vi "BioFeedback17(Queue).vi"(7 "Frames Per Second":dbl=30.0, 9 "Start Trial":bool, 11 "End Trial":bool, 12 "Data Directory":path=path "C:/Users/Tinggroup/Desktop/VRMuscleActivationVisualizer/LabviewFiles/Data/Test", 13 "File Name":string="Test") -> ()   [LabVIEW 2016]
uses:
  customSubVIs/Control 1.ctl
  <vilib>/Utility/file.llb/Write Delimited Spreadsheet (DBL).vi
  <vilib>/Waveform/WDTFileIO.llb/Export Waveforms To Spreadsheet File (1D).vi
  <vilib>/Utility/file.llb/Write Delimited Spreadsheet (I64).vi
  <vilib>/Utility/error.llb/DialogType.ctl
panel:
  out "error out 3":errorcluster
  out "Raw Trial Data Wfm 2":waveform(dbl)[](graph)
  out "Terminate":bool=TRUE
  out "Waveform":waveform(dbl)
  out "Notes":T1(array[cluster])
  in  "Mark":bool
  out "error out 2":errorcluster
  out "error out":errorcluster
  out "MVC Buffer Index":dbl=3.0
  in  "DisplayDataPath":path
  in  "FilteredDataPath":path
  in  "RawDataPath":path
  in  "MVC Number":dbl=1.0
  out "Save MVC":bool
  out "Display Buffer":dbl[][](array[numeric])
  out "Display Buffer Index":dbl=3.0
  out "FilteredTrialData Display Channel":waveform(dbl)(graph)
  out "Raw Trial Data Display Channel":waveform(dbl)(graph)
  out "EndProcessTic":u32
  out "StartProcessTic":u32
  out "EndRecordTic":u32
  out "startRecordTic":u32
  out "Start UI":timestamp
  out "UI Elapsed Time":u32
  out "End UI":timestamp
  out "Process Elapsed Time":u32
  out "Record Elapsed Time":u32
  out "FilteredTrialData":waveform(dbl)[](graph)
  out "FilteredAndRectified":waveform(dbl)[](graph) caption="Filtered and Rectified"
  out "FilteredDataArray":waveform(dbl)[](array[waveform])
  in  "DisplayChannel":dbl
  out "DisplayTrialData":T2
  out "DisplayValueByChannel":dbl[](array[numeric])
  out "MVCBufferSize":dbl
  in  "MVC Window Size (s)":dbl=0.5
  out "MVC Buffer":dbl[][](array[numeric])
  out "GetMaxStartTime":timestamp
  in  "SecondsToAcquireMax":dbl=3.0
  out "MVCArray":dbl[](array[numeric])
  out "RawTrialData":waveform(dbl)[](array[waveform])
  in  "UI Ampl Error Path":path=path "C:/Users/Tinggroup/Desktop/VRMuscleActivationVisualizer/VRBiofeedback_v2/assets/BiofeedbackAmplitudeError.txt"
  out "DisplayActivation":dbl
  out "Get MVC":bool
  in  "resetMax":bool
  in  "startGetMax":bool
  in  "Amplitude Error":dbl
  in  "UI Data Path":path=path "C:/Users/Tinggroup/Desktop/VRMuscleActivationVisualizer/VRBiofeedback_v2/assets/LeftEMGData.txt"
  in  "EMG Input Device\nProduct Type":string="USB-6009"
  out "DisplayBarActivation":dbl(slide) caption="Left" max=1.0 scale=0.0..100.0
  out "NormalizedSignal8":dbl[](graph)
  out "NormalizedSignal7":dbl[](graph)
  out "NormalizedSignal6":dbl[](graph)
  out "NormalizedSignal5":dbl[](graph)
  out "NormalizedSignal4":dbl[](graph)
  out "NormalizedSignal3":dbl[](graph)
  out "NormalizedSignal2":dbl[](graph)
  out "NormalizedSignal1":dbl[](graph)
  out "Raw Trial Data Wfm":waveform(dbl)[](graph)
  in  "UI Percent Path":path=path "C:/Users/Tinggroup/Desktop/VRMuscleActivationVisualizer/VRBiofeedback_v2/assets/BiofeedbackTargetPercentage.txt"
  in  "Target Percentage":dbl=10.0
  out "Trial In Progress":bool
  in  "Lower Cut-Off":dbl=20.0
  in  "Upper Cut-Off":dbl=300.0
  out "raw data":dynamicdata(graph)
  out "DisplayBufferSize":dbl
  out "Samples per frame":dbl
  out "Reset":bool=TRUE
  in  "Display Window Size (s)":dbl=0.5
  in  "Sample rate (Hz)":dbl=2000.0
  in  "End Program":bool
  # "Data To Be Saved (Not including Max Data)"
  # "Performance Metrics"
  # "Saving Trial Data"
  # "Small Window"
  # "Scale Max"
  # "Filter and Process Parameters"
  # "MVC Buffer"
  # "Set Target"
  # "Display Parameters"
  # "Changes are made instantly and cause moving average to reset to zero"
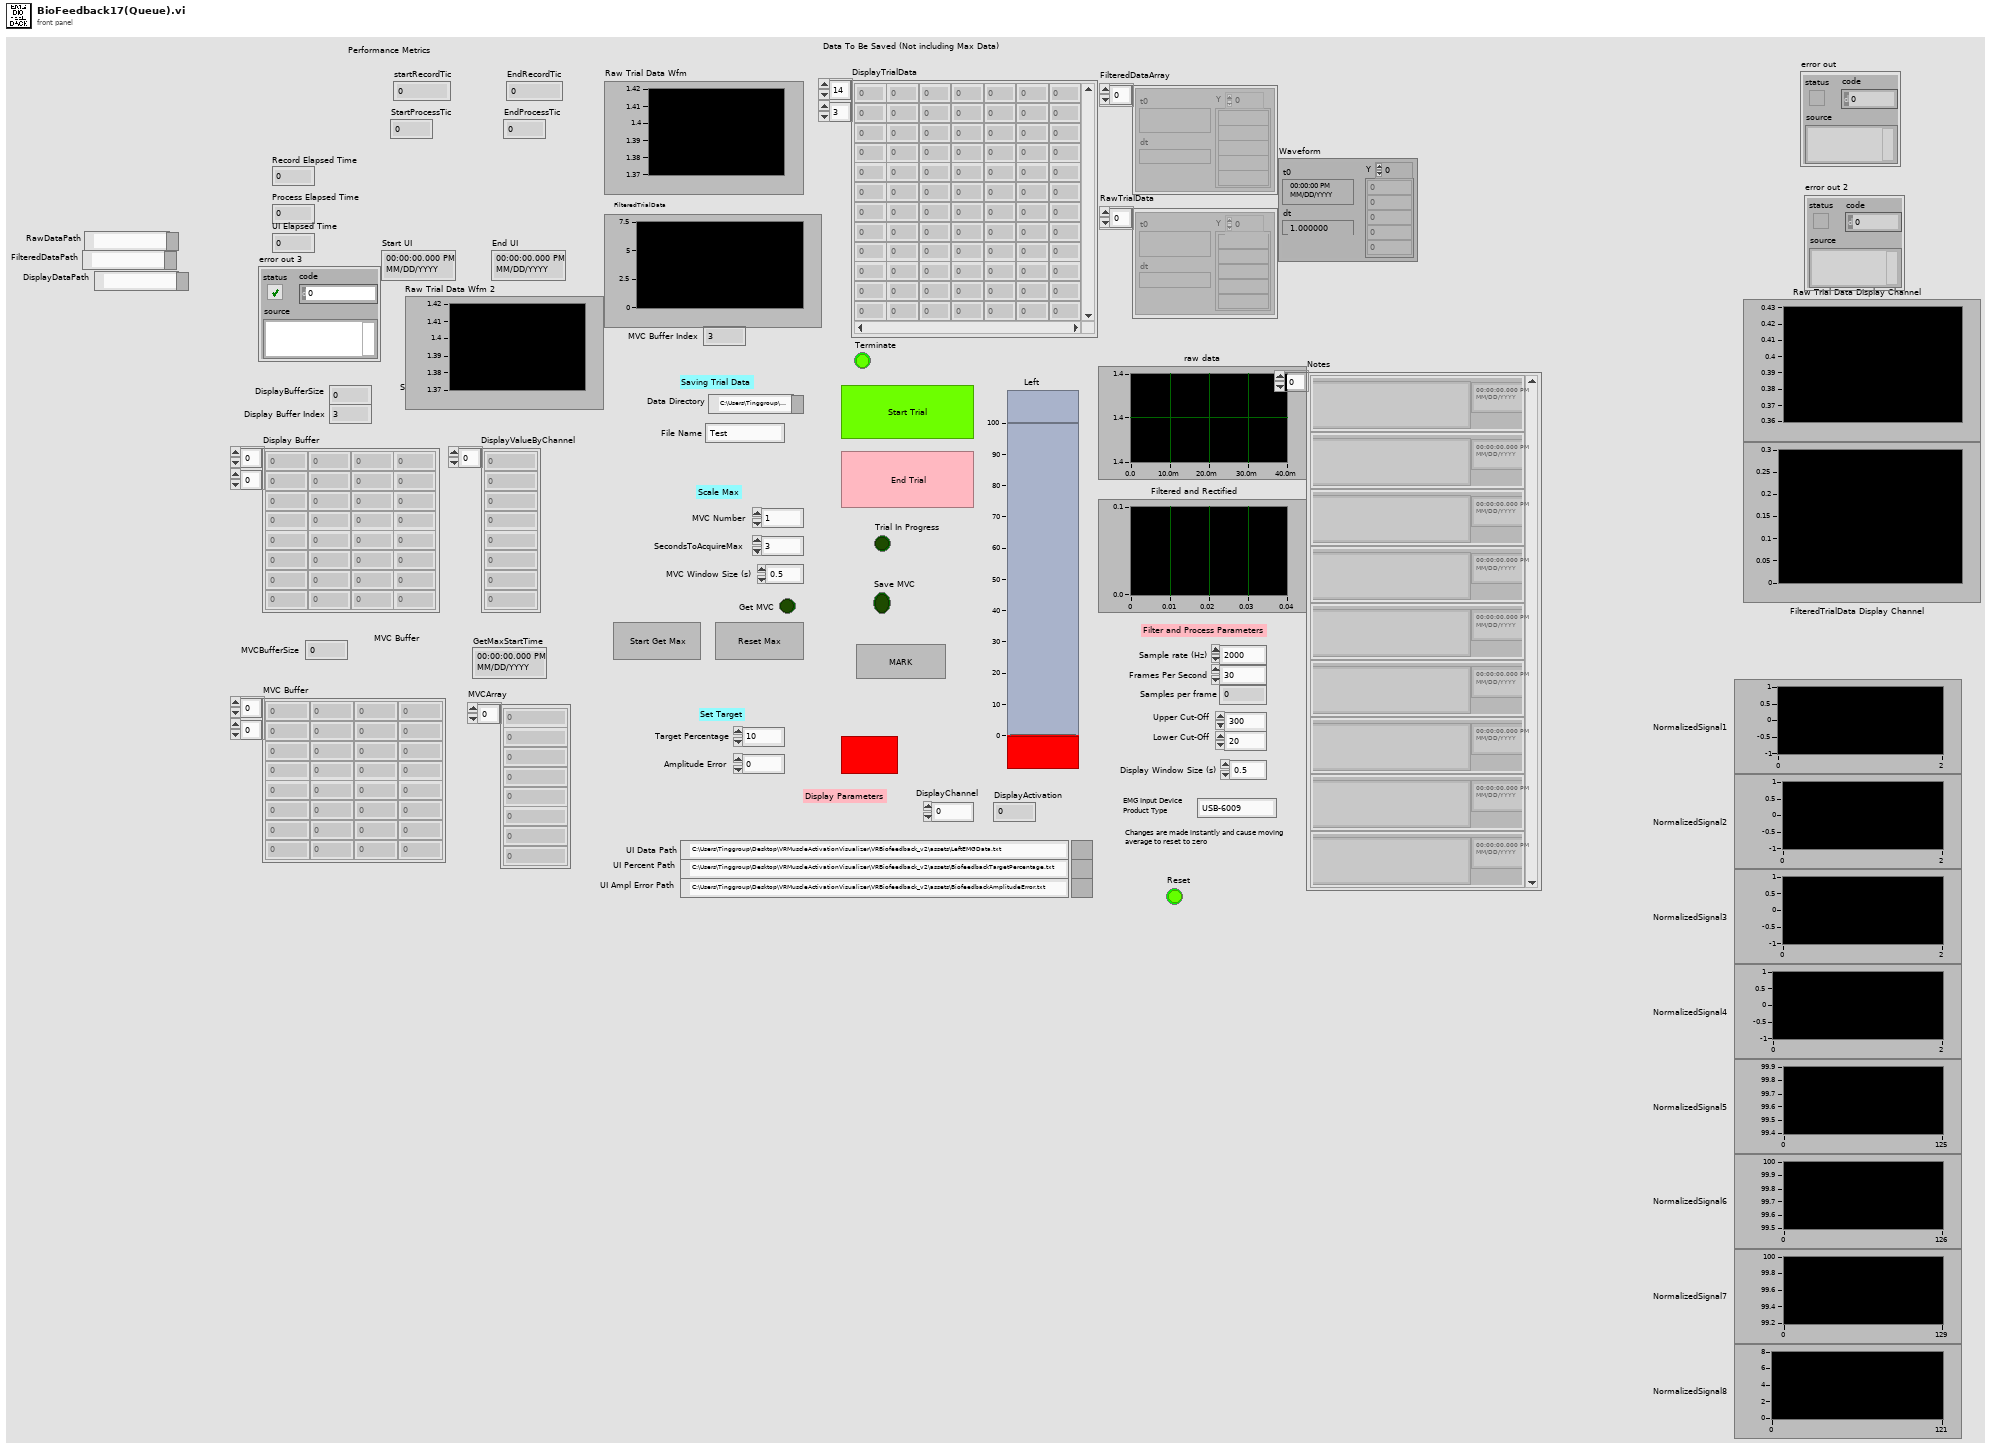
[diagram p1: front panel]
types:
  T1 = cluster{"Time Stamp":timestamp, "String":string}[]
  T2 = typedef "Control 1.ctl" = dbl[][]
  T3 = cluster{"seconds since 1Jan1904":timestamp, string}
  T4 = typedef "DialogType.ctl" = u16
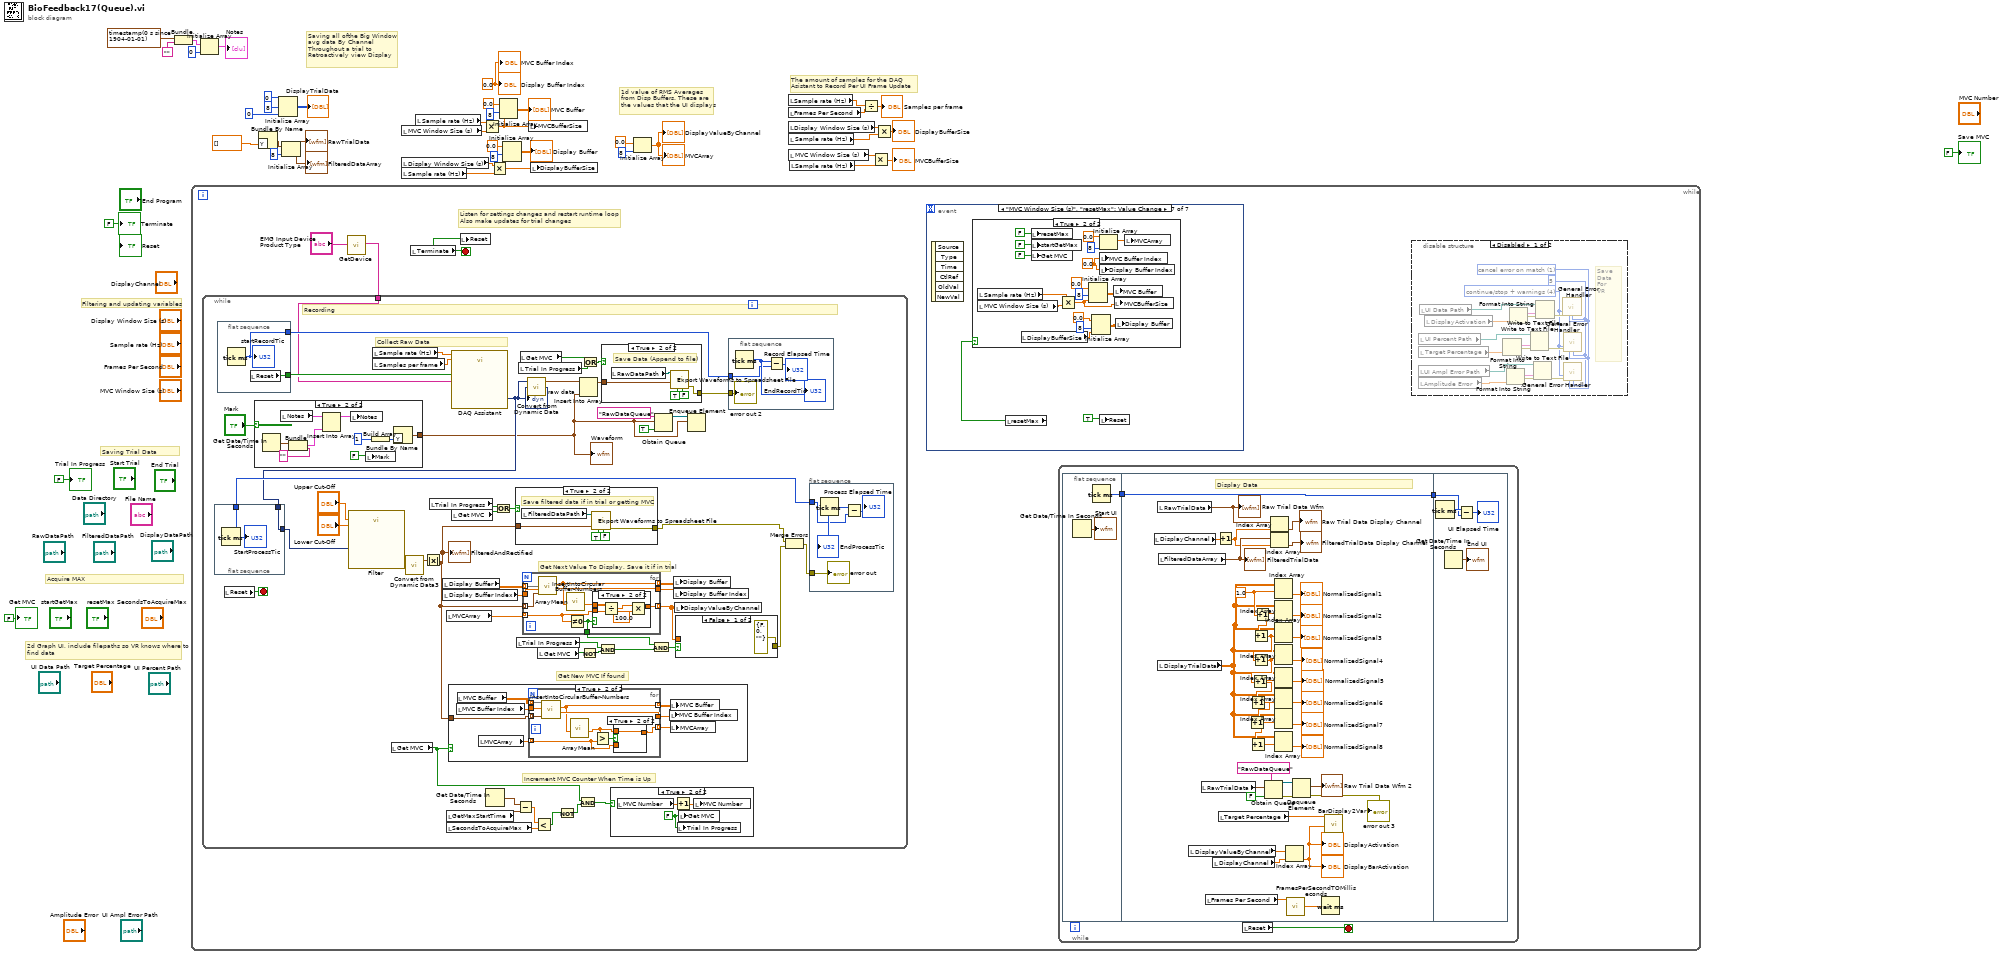
[diagram p0: block diagram]
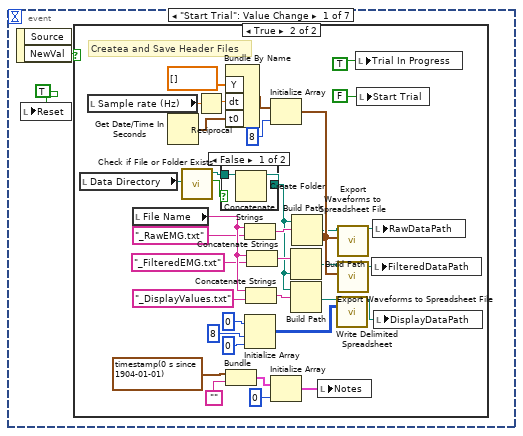
[diagram p3: hidden frame]
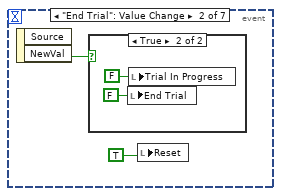
[diagram p6: hidden frame]
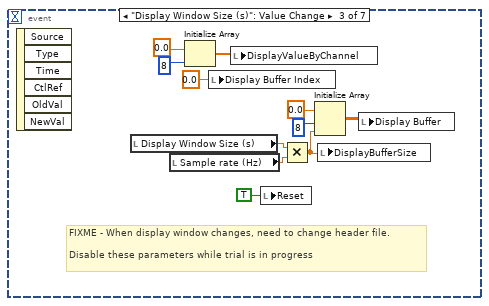
[diagram p8: hidden frame]
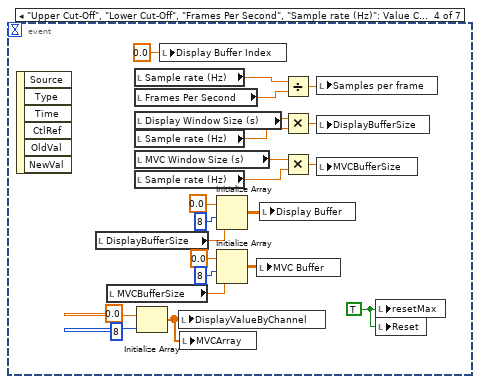
[diagram p9: hidden frame]
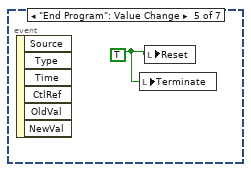
[diagram p10: hidden frame]
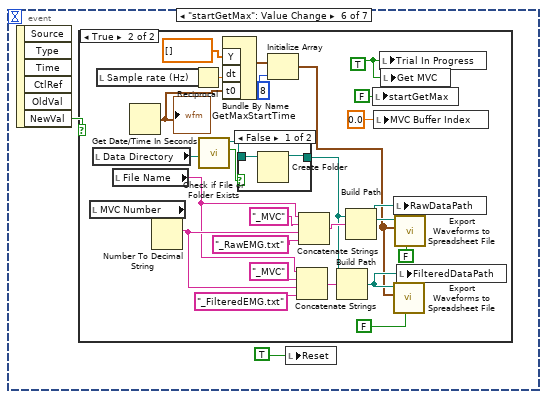
[diagram p11: hidden frame]
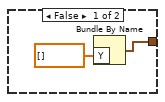
[diagram p15: hidden frame]
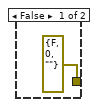
[diagram p16: hidden frame]
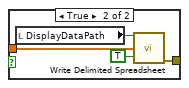
[diagram p17: hidden frame]
diagram:
  w13 = 0.0 ("Display Buffer Index")
  # "The amount of samples for the DAQ Asistant to Record Per UI Frame Update"
  # "Saving all ofthe Big Window \navg data By Channel\nThroughout a trial to \nRetroactively view Display"
  # "1d value of RMS Averages\nfrom Disp Buffers. These are\nthe values that the UI displays"
  # "Acquire MAX"
  # "Filtering and updating variables"
  # "Saving Trial Data"
  # "2d Graph UI, include filepaths so VR knows where to find data"
  n1 = Bundle(timestamp(0 s since 1904-01-01), "") -> (w12:cluster{timestamp, string})  [unwired: 1 in]
  n2 = while {
    stop <- w43 stop-if-true
    # "Listen for settings changes and restart runtime loop\nAlso make updates for trial changes"
    n3 = call "GetDevice.vi"("EMG Input Device\nProduct Type"="EMG Input Device\nProduct Type") -> ("DAQmx Device Name"=w45:tag)  [unwired: 10 in]
    n4 = while {
      tunnel: w45 -> [w247]
      stop <- w286 stop-if-true
      # "Recording"
      # "Collect Raw Data"
      # "Increment MVC Counter When Time is Up"
      # "Get New MVC If found"
      # "Get Next Value To Display, Save it if in trial"
      n5 = flat-sequence {
        tunnel: [w315] -> w258
        tunnel: [w314] -> w241
        tunnel: w240 -> [w314]
        frame #0 {
          n6 = Tick Count (ms)() -> (millisecond timer value=w315:u32)
          "StartProcessTic" <- w315
        }
      }
      n7 = flat-sequence {
        tunnel: [w303] -> w252
        tunnel: [w302] -> w251
        frame #0 {
          n8 = Tick Count (ms)() -> (millisecond timer value=w302:u32)
          "startRecordTic" <- w302
          n9 = local read "Reset"() -> (w303:bool)
        }
      }
      n10 = local read "Reset"() -> (w286:bool)
      n11 = case shown="True" "Mark" {
        tunnel: [w287 w290] -> w236
        frame False {
          n12 = Bundle By Name("Y"=dbl[] []) -> (w287:waveform(dbl))  [unwired: 1 in]
        }
        frame True {
          n13 = Get Date/Time In Seconds() -> (seconds since 1Jan1904=w296:timestamp)
          n14 = local read "Notes"() -> (w293:T1)
          n15 = Bundle("seconds since 1Jan1904"=w296, "") -> (w292:T3)  [unwired: 1 in]
          n16 = Insert Into Array(array=w293, new element=w292) -> (w294:T1)  [unwired: 1 in]
          n17 = local write "Notes"(w294) -> ()
          n18 = local write "Mark"(FALSE) -> ()
          n19 = Build Array(1) -> (w291:i32[])
          n20 = Bundle By Name("Y"=w291) -> (w290:waveform(i32))  [unwired: 1 in]
        }
      }
      "Waveform" <- w236
      n21 = call "Filter"("Lower Cut-Off"="Lower Cut-Off", "Upper Cut-Off"="Upper Cut-Off", "Signal"=w241) -> ("Filtered Signal"=w242:dynamicdata)  [unwired: 7 in, 1 out]
      n22 = local read "Sample rate (Hz)"() -> (w253:dbl)
      n23 = local read "Samples per frame"() -> (w254:dbl)
      n24 = local read "Get MVC"() -> (w279:bool)
      n25 = call "Convert from Dynamic Data3"("Dynamic Data Type"=w242) -> ("Array of Waveform"=w259:waveform(dbl)[])  [unwired: 3 in]
      n26 = Absolute Value(x=w259) -> (abs(x)=w274:waveform(dbl)[])
      "FilteredAndRectified" <- w274
      n27 = local read "Trial In Progress"() -> (w262:bool)
      n28 = local read "Display Buffer"() -> (w265:dbl[][])
      n29 = local read "Display Buffer Index"() -> (w266:dbl)
      n30 = local read "MVCArray"() -> (w269:dbl[])
      n31 = local read "GetMaxStartTime"() -> (w273:timestamp)
      n32 = local read "SecondsToAcquireMax"() -> (w270:dbl)
      n33 = case shown="True" w279 {
        tunnel: w274 -> [_ w328]
        frame False {
        }
        frame True {
          n34 = local read "MVC Buffer Index"() -> (w330:dbl)
          n35 = local read "MVC Buffer"() -> (w329:dbl[][])
          n36 = local read "MVCArray"() -> (w327:dbl[])
          n37 = for {
            tunnel: w329 -> [w339] mode=indexing
            tunnel: w330 -> [w331]
            tunnel: [w338] -> w324
            tunnel: w328 -> [w337] mode=indexing
            tunnel: w327 -> [w333] mode=indexing
            tunnel: [w332] -> w326 mode=indexing
            tunnel: [w334] -> w325 mode=indexing
            n38 = call "InsertIntoCircularBuffer-Numbers.vi"("NewElements"=w337, "StartIndex"=w331, "Buffer"=w339) -> ("New Start Index"=w338:dbl, "UpdatedBuffer"=w334:dbl[])  [unwired: 7 in]
            n39 = call "ArrayMean.vi"("Array"=w334) -> ("Mean"=w335:dbl)  [unwired: 10 in]
            n40 = Greater?(x=w335, y=w333) -> (0:w336:bool)
            n41 = case shown="True" w336 {
              tunnel: w335 -> [_ w341]
              tunnel: [w340 w341] -> w332
              tunnel: w333 -> [w340 _]
              frame False {
              }
              frame True {
              }
            }
          }
          n42 = local write "MVC Buffer Index"(w324) -> ()
          n43 = local write "MVC Buffer"(w325) -> ()
          n44 = local write "MVCArray"(w326) -> ()
        }
      }
      n45 = call "DAQ Assistant"("rate"=w253, "number of samples"=w254, "stop (F)"=w252, "device name"=w247) -> ("data"=w240:dynamicdata)  [unwired: 12 in, 3 out]
      "raw data" <- w240
      n46 = local read "Get MVC"() -> (w264:bool)
      n47 = Get Date/Time In Seconds() -> (seconds since 1Jan1904=w272:timestamp)
      n48 = Or(x=w262, y=w264) -> (x .or. y?=w263:bool)
      n49 = case shown="True" w263 {
        tunnel: w274 -> [_ w359]
        tunnel: [errorcluster {"status"=FALSE, "code"=0, "source"=""} ("error out") w358] -> w249
        frame False {
        }
        frame True {
          # "Save filtered data if in trial or getting MVC"
          n50 = local read "FilteredDataPath"() -> (w360:path)
          n51 = call-poly <vilib>:"Export Waveforms to Spreadsheet File.vi"("header? (write header:T)"=FALSE, "append to file? (new file:F)"=TRUE, "waveforms"=w359, "file path (dialog if empty)"=w360) -> ("error out"=w358:errorcluster)  [unwired: 6 in, 1 out]
        }
      }
      n52 = local read "Trial In Progress"() -> (w284:bool)
      n53 = Subtract(x=w272, y=w273) -> (x-y=w271:dbl)
      n54 = local read "Trial In Progress"() -> (w255:bool)
      n55 = local read "Get MVC"() -> (w256:bool)
      n56 = for {
        tunnel: w265 -> [w350] mode=indexing
        tunnel: w274 -> [w343] mode=indexing
        tunnel: w266 -> [w349]
        tunnel: [w347] -> w267 mode=indexing
        tunnel: [w348] -> w268
        tunnel: w269 -> [w345] mode=indexing
        tunnel: [w344] -> w278 mode=indexing
        tunnel: [w342] -> w281
        n57 = call "InsertIntoCircularBuffer-Numbers.vi"("NewElements"=w343, "StartIndex"=w349, "Buffer"=w350) -> ("New Start Index"=w348:dbl, "UpdatedBuffer"=w347:dbl[])  [unwired: 7 in]
        n58 = call "ArrayMean.vi"("Array"=w347) -> ("Mean"=w346:dbl)  [unwired: 10 in]
        n59 = Not Equal To 0?(x=w345) -> (x != 0?=w342:bool)
        n60 = case shown="True" w342 {
          tunnel: w346 -> [_ w355]
          tunnel: w345 -> [_ w356]
          tunnel: [0.0 w354] -> w344
          frame False {
          }
          frame True {
            n61 = Divide(x=w355, y=w356) -> (x/y=w353:dbl)
            n62 = Multiply(x=w353, y=100.0) -> (x*y=w354:dbl)
          }
        }
      }
      n63 = call "Convert from Dynamic Data"("Dynamic Data Type"=w240) -> ("Array of Waveform"=w244:waveform(dbl)[])  [unwired: 3 in]
      n64 = Less?(x=w271, y=w270) -> (x < y?=w275:bool)
      n65 = local read "Get MVC"() -> (w282:bool)
      n66 = Not(x=w275) -> (.not. x?=w276:bool)
      n67 = And(x=w279, y=w276) -> (x .and. y?=w277:bool)
      n68 = Insert Into Array(array=w244, new element=w236) -> (w243:waveform(dbl)[])  [unwired: 1 in]
      n69 = Not(x=w282) -> (.not. x?=w283:bool)
      n70 = Or(x=w256, y=w255) -> (x .or. y?=w257:bool)
      n71 = And(x=w284, y=w283) -> (x .and. y?=w285:bool)
      n72 = case shown="True" w257 {
        tunnel: w243 -> [_ w307]
        tunnel: [errorcluster {"status"=FALSE, "code"=0, "source"=""} ("error out") w305] -> w246
        frame False {
        }
        frame True {
          # "Save Data (Append to file)"
          n73 = local read "RawDataPath"() -> (w306:path)
          n74 = call-poly <vilib>:"Export Waveforms to Spreadsheet File.vi"("header? (write header:T)"=FALSE, "append to file? (new file:F)"=TRUE, "waveforms"=w307, "file path (dialog if empty)"=w306) -> ("error out"=w305:errorcluster)  [unwired: 6 in, 1 out]
        }
      }
      n75 = case shown="True" w277 {
        frame False {
        }
        frame True {
          w321 = FALSE ("Get MVC")
          n76 = local read "MVC Number"() -> (w322:dbl)
          n77 = Increment(x=w322) -> (x+1=w323:dbl)
          n78 = local write "Trial In Progress"(w321) -> ()
          n79 = local write "Get MVC"(w321) -> ()
          n80 = local write "MVC Number"(w323) -> ()
        }
      }
      n81 = And(x=w281, y=w285) -> (x .and. y?=w280:bool)
      n82 = Obtain Queue(name (unnamed)="RawDataQueue", element data type=w236, create if not found? (T)=TRUE) -> (queue out=w237:refnum<queue>)  [unwired: 2 in, 2 out]
      n83 = local write "Display Buffer"(w267) -> ()
      n84 = local write "Display Buffer Index"(w268) -> ()
      n85 = local write "DisplayValueByChannel"(w278) -> ()
      n86 = case shown="False" w280 {
        tunnel: w278 -> [_ w319]
        tunnel: [errorcluster {"status"=FALSE, "code"=0, "source"=""} ("error out") w317] -> w250
        frame False {
        }
        frame True {
          n87 = local read "DisplayDataPath"() -> (w318:path)
          n88 = call-poly <vilib>:"Write Delimited Spreadsheet.vi"("file path (dialog if empty)"=w318, "1D data"=w319, "append to file? (new file:F)"=TRUE) -> ("error out"=w317:errorcluster)  [unwired: 11 in, 1 out]
        }
      }
      n89 = Enqueue Element(queue=w237, element=w236) -> ()  [unwired: 2 in, 3 out]
      n90 = flat-sequence {
        tunnel: w251 -> [w299]
        tunnel: w246 -> [w298]
        frame #0 {
          n91 = Tick Count (ms)() -> (millisecond timer value=w301:u32)
          "EndRecordTic" <- w301
          n92 = Subtract(x=w301, y=w299) -> (x-y=→"Record Elapsed Time":u32)
          "error out 2" <- w298
        }
      }
      n93 = Merge Errors(w249, w250) -> (w248:errorcluster)
      n94 = flat-sequence {
        tunnel: w258 -> [w311]
        tunnel: w248 -> [w310]
        frame #0 {
          n95 = Tick Count (ms)() -> (millisecond timer value=w312:u32)
          "EndProcessTic" <- w312
          n96 = Subtract(x=w312, y=w311) -> (x-y=→"Process Elapsed Time":u32)
          "error out" <- w310
        }
      }
    }
    n97 = local read "Terminate"() -> (w43:bool)
    n98 = local write "Reset"(w43) -> ()
    n99 = event shown="[6] \"MVC Window Size (s)\", \"resetMax\": Value Change" {
      selector: _ -> [_ _ _ _ _ _ _]
      dyn-events: _ -> [_ _ _ _ _ _ _]
      timeout: _ -> [_ _ _ _ _ _ _]
      event "Start Trial": Value Change {
        n100 = event-data() -> ("NewVal"=w111:bool)  [unwired: 1 in, 1 out]
        n101 = local write "Reset"(TRUE ("Trial In Progress")) -> ()
        n102 = case shown="True" w111 {
          frame False {
          }
          frame True {
            # "Createa and Save Header Files"
            n103 = local read "Data Directory"() -> (w130:path)
            n104 = local read "Sample rate (Hz)"() -> (w139:dbl)
            n105 = local read "File Name"() -> (w136:string)
            n106 = Get Date/Time In Seconds() -> (seconds since 1Jan1904=w137:timestamp)
            n107 = call <vilib>:"Check if File or Folder Exists.vi"("path"=w130) -> ("file or folder exists?"=w129:bool, "dup path"=w128:path)  [unwired: 8 in, 1 out]
            n108 = Reciprocal(x=w139) -> (1/x=w138:dbl)
            n109 = case shown="False" w129 {
              tunnel: [w144 w146] -> w127
              tunnel: w128 -> [w145 w146]
              frame False {
                n110 = Create Folder(path (use dialog)=w145) -> (created path=w144:path)  [unwired: 2 in, 2 out]
              }
              frame True {
              }
            }
            n111 = Bundle By Name("Y"=dbl[] [], "dt"=w138, "t0"=w137) -> (w142:waveform(dbl))  [unwired: 1 in]
            n112 = Bundle(timestamp(0 s since 1904-01-01), "") -> (w116:cluster{timestamp, string})  [unwired: 1 in]
            n113 = Concatenate Strings(w136, "_RawEMG.txt" ("string")) -> (w131:string)
            n114 = Initialize Array(0, 8 ("dimension size"), 0 ("dimension size")) -> (w118:i32[][])
            n115 = Concatenate Strings(w136, "_DisplayValues.txt" ("string")) -> (w134:string)
            n116 = Concatenate Strings(w136, "_FilteredEMG.txt" ("string")) -> (w132:string)
            n117 = Initialize Array(w142, 8 ("dimension size")) -> (w126:waveform(dbl)[])
            n118 = Initialize Array(w116, 0 ("dimension size")) -> (w112:cluster{timestamp, string}[])
            n119 = Build Path(base path=w127, name or relative path=w132) -> (appended path=w123:path)
            n120 = Build Path(base path=w127, name or relative path=w134) -> (appended path=w122:path)
            n121 = Build Path(base path=w127, name or relative path=w131) -> (appended path=w124:path)
            n122 = local write "Notes"(w112) -> ()
            n123 = call-poly <vilib>:"Write Delimited Spreadsheet.vi"("file path (dialog if empty)"=w122, "2D data"=w118) -> ()  [unwired: 12 in, 2 out]
            n124 = call-poly <vilib>:"Export Waveforms to Spreadsheet File.vi"("waveforms"=w126, "file path (dialog if empty)"=w124) -> ()  [unwired: 8 in, 2 out]
            n125 = call-poly <vilib>:"Export Waveforms to Spreadsheet File.vi"("waveforms"=w126, "file path (dialog if empty)"=w123) -> ()  [unwired: 8 in, 2 out]
            n126 = local write "Trial In Progress"(TRUE ("Trial In Progress")) -> ()
            n127 = local write "Start Trial"(FALSE ("Start Trial")) -> ()
            n128 = local write "FilteredDataPath"(w123) -> ()
            n129 = local write "RawDataPath"(w124) -> ()
            n130 = local write "DisplayDataPath"(w122) -> ()
          }
        }
      }
      event "End Trial": Value Change {
        n131 = event-data() -> ("NewVal"=w148:bool)  [unwired: 1 in, 1 out]
        n132 = case shown="True" w148 {
          frame False {
          }
          frame True {
            n133 = local write "End Trial"(FALSE ("End Trial")) -> ()
            n134 = local write "Trial In Progress"(FALSE ("Trial In Progress")) -> ()
          }
        }
        n135 = local write "Reset"(TRUE ("Reset Data Acquisition\nAnd UI Updating")) -> ()
      }
      event "Display Window Size (s)": Value Change {
        # "FIXME - When display window changes, need to change header file.\n\nDisable these parameters while trial is in progress"
        n136 = event-data() -> ()  [unwired: 1 in, 6 out]
        n137 = local read "Display Window Size (s)"() -> (w153:dbl)
        n138 = local read "Sample rate (Hz)"() -> (w152:dbl)
        n139 = Initialize Array(0.0 ("element"), 8 ("dimension size")) -> (w158:dbl[])
        n140 = local write "Display Buffer Index"(0.0 ("Display Buffer Index")) -> ()
        n141 = local write "DisplayValueByChannel"(w158) -> ()
        n142 = local write "Reset"(TRUE ("Reset")) -> ()
        n143 = Multiply(x=w153, y=w152) -> (x*y=w151:dbl)
        n144 = Initialize Array(0.0 ("element"), 8 ("dimension size"), w151) -> (w154:dbl[][])
        n145 = local write "DisplayBufferSize"(w151) -> ()
        n146 = local write "Display Buffer"(w154) -> ()
      }
      event "Upper Cut-Off", "Lower Cut-Off", "Frames Per Second", "Sample rate (Hz)": Value Change {
        w168 = TRUE
        n147 = event-data() -> ()  [unwired: 1 in, 6 out]
        n148 = local read "DisplayBufferSize"() -> (w173:dbl)
        n149 = local read "MVCBufferSize"() -> (w165:dbl)
        n150 = local read "Sample rate (Hz)"() -> (w183:dbl)
        n151 = local read "Frames Per Second"() -> (w182:dbl)
        n152 = local read "Display Window Size (s)"() -> (w180:dbl)
        n153 = local read "Sample rate (Hz)"() -> (w179:dbl)
        n154 = local read "MVC Window Size (s)"() -> (w178:dbl)
        n155 = local read "Sample rate (Hz)"() -> (w177:dbl)
        n156 = Initialize Array(0.0 ("element"), 8 ("dimension size")) -> (w167:dbl[])
        n157 = local write "Display Buffer Index"(0.0 ("Display Buffer Index")) -> ()
        n158 = local write "DisplayValueByChannel"(w167) -> ()
        n159 = local write "MVCArray"(w167) -> ()
        n160 = Initialize Array(0.0 ("element"), 8 ("dimension size"), w173) -> (w171:dbl[][])
        n161 = Initialize Array(0.0 ("element"), 8 ("dimension size"), w165) -> (w163:dbl[][])
        n162 = local write "MVC Buffer"(w163) -> ()
        n163 = local write "Display Buffer"(w171) -> ()
        n164 = Divide(x=w183, y=w182) -> (x/y=w181:dbl)
        n165 = Multiply(x=w180, y=w179) -> (x*y=w175:dbl)
        n166 = Multiply(x=w178, y=w177) -> (x*y=w176:dbl)
        n167 = local write "Samples per frame"(w181) -> ()
        n168 = local write "DisplayBufferSize"(w175) -> ()
        n169 = local write "MVCBufferSize"(w176) -> ()
        n170 = local write "resetMax"(w168) -> ()
        n171 = local write "Reset"(w168) -> ()
      }
      event "End Program": Value Change {
        w184 = TRUE
        n172 = event-data() -> ()  [unwired: 1 in, 6 out]
        n173 = local write "Terminate"(w184) -> ()
        n174 = local write "Reset"(w184) -> ()
      }
      event "startGetMax": Value Change {
        n175 = event-data() -> ("NewVal"=w186:bool)  [unwired: 1 in, 5 out]
        n176 = case shown="True" w186 {
          frame False {
          }
          frame True {
            w191 = TRUE ("Trial In Progress")
            n177 = local read "MVC Number"() -> (w205:dbl)
            n178 = local read "Data Directory"() -> (w209:path)
            n179 = local read "Sample rate (Hz)"() -> (w201:dbl)
            n180 = local read "File Name"() -> (w198:string)
            n181 = Get Date/Time In Seconds() -> (seconds since 1Jan1904=w199:timestamp)
            "GetMaxStartTime" <- w199
            n182 = Number To Decimal String(number=w205) -> (decimal integer string=w208:string)  [unwired: 1 in]
            n183 = Reciprocal(x=w201) -> (1/x=w200:dbl)
            n184 = call <vilib>:"Check if File or Folder Exists.vi"("path"=w209) -> ("file or folder exists?"=w206:bool, "dup path"=w213:path)  [unwired: 8 in, 1 out]
            n185 = Bundle By Name("Y"=dbl[] [], "dt"=w200, "t0"=w199) -> (w203:waveform(dbl))  [unwired: 1 in]
            n186 = case shown="False" w206 {
              tunnel: w213 -> [w215 w216]
              tunnel: [w214 w216] -> w195
              frame False {
                n187 = Create Folder(path (use dialog)=w215) -> (created path=w214:path)  [unwired: 2 in, 2 out]
              }
              frame True {
              }
            }
            n188 = Initialize Array(w203, 8 ("dimension size")) -> (w190:waveform(dbl)[])
            n189 = Concatenate Strings(w198, "_MVC" ("string"), w208, "_FilteredEMG.txt" ("string")) -> (w211:string)
            n190 = Concatenate Strings(w198, "_MVC" ("string"), w208, "_RawEMG.txt" ("string")) -> (w210:string)
            n191 = Build Path(base path=w195, name or relative path=w211) -> (appended path=w193:path)
            n192 = Build Path(base path=w195, name or relative path=w210) -> (appended path=w204:path)
            n193 = local write "startGetMax"(FALSE ("Start Trial")) -> ()
            n194 = local write "MVC Buffer Index"(0.0 ("MVC Buffer Indes")) -> ()
            n195 = local write "Trial In Progress"(w191) -> ()
            n196 = local write "Get MVC"(w191) -> ()
            n197 = local write "RawDataPath"(w204) -> ()
            n198 = call-poly <vilib>:"Export Waveforms to Spreadsheet File.vi"("append to file? (new file:F)"=FALSE, "waveforms"=w190, "file path (dialog if empty)"=w193) -> ()  [unwired: 7 in, 2 out]
            n199 = call-poly <vilib>:"Export Waveforms to Spreadsheet File.vi"("append to file? (new file:F)"=FALSE, "waveforms"=w190, "file path (dialog if empty)"=w204) -> ()  [unwired: 7 in, 2 out]
            n200 = local write "FilteredDataPath"(w193) -> ()
          }
        }
        n201 = local write "Reset"(TRUE ("Reset Data Acquisition\nAnd UI Updating")) -> ()
      }
      event "MVC Window Size (s)", "resetMax": Value Change {
        n202 = event-data() -> ()  [unwired: 1 in, 6 out]
        n203 = local read "resetMax"() -> (w217:bool)
        n204 = case shown="True" w217 {
          frame False {
          }
          frame True {
            w229 = 0.0 ("MVC Buffer Index")
            n205 = local read "Sample rate (Hz)"() -> (w221:dbl)
            n206 = local read "MVC Window Size (s)"() -> (w220:dbl)
            n207 = local read "DisplayBufferSize"() -> (w223:dbl)
            n208 = local write "resetMax"(FALSE ("endGetMax")) -> ()
            n209 = local write "startGetMax"(FALSE ("startGetMax")) -> ()
            n210 = local write "Get MVC"(FALSE ("Acquiring Max")) -> ()
            n211 = Multiply(x=w221, y=w220) -> (x*y=w219:dbl)
            n212 = Initialize Array(0.0 ("element"), 8 ("dimension size"), w219) -> (w226:dbl[][])
            n213 = Initialize Array(0.0 ("element"), 8 ("dimension size"), w223) -> (w222:dbl[][])
            n214 = Initialize Array(0.0 ("element"), 8 ("dimension size")) -> (w230:dbl[])
            n215 = local write "MVC Buffer Index"(w229) -> ()
            n216 = local write "Display Buffer Index"(w229) -> ()
            n217 = local write "MVC Buffer"(w226) -> ()
            n218 = local write "MVCBufferSize"(w219) -> ()
            n219 = local write "Display Buffer"(w222) -> ()
            n220 = local write "MVCArray"(w230) -> ()
          }
        }
        n221 = local write "Reset"(TRUE ("Reset Data Acquisition\nAnd UI Updating")) -> ()
      }
    }
    n222 = while {
      stop <- w64 stop-if-true
      n223 = flat-sequence {
        tunnel: [w68] -> w66
        tunnel: [w105] -> w65
        tunnel: w66 -> [w105]
        tunnel: w65 -> [w106]
        frame #0 {
          n224 = Get Date/Time In Seconds() -> (seconds since 1Jan1904=→"Start UI":timestamp)
          n225 = Tick Count (ms)() -> (millisecond timer value=w68:u32)
        }
        frame #1 {
          w79 = 1.0 ("x")
          # "Display Data"
          n226 = local read "DisplayChannel"() -> (w100:dbl)
          n227 = local read "RawTrialData"() -> (w95:waveform(dbl)[])
          "Raw Trial Data Wfm" <- w95
          n228 = local read "DisplayTrialData"() -> (w78:T2)
          n229 = local read "FilteredDataArray"() -> (w99:waveform(dbl)[])
          "FilteredTrialData" <- w99
          n230 = local read "DisplayValueByChannel"() -> (w104:dbl[])
          n231 = local read "RawTrialData"() -> (w72:waveform(dbl)[])
          n232 = local read "Frames Per Second"() -> (w102:dbl)
          n233 = local read "DisplayChannel"() -> (w101:dbl)
          n234 = Increment(x=w100) -> (x+1=w98:dbl)
          n235 = local read "Target Percentage"() -> (w77:dbl)
          n236 = Increment(x=w79) -> (x+1=w80:dbl)
          n237 = Increment(x=w80) -> (x+1=w81:dbl)
          n238 = Increment(x=w81) -> (x+1=w82:dbl)
          n239 = Increment(x=w82) -> (x+1=w83:dbl)
          n240 = Increment(x=w83) -> (x+1=w84:dbl)
          n241 = Increment(x=w84) -> (x+1=w85:dbl)
          n242 = Increment(x=w85) -> (x+1=w86:dbl)
          n243 = Obtain Queue(name (unnamed)="RawDataQueue", element data type=w72, create if not found? (T)=FALSE) -> (queue out=w75:refnum<queue>, error out=w74:errorcluster)  [unwired: 2 in, 1 out]
          n244 = Index Array(array=w95, index=w98) -> (element=→"Raw Trial Data Display Channel":waveform(dbl))
          n245 = Index Array(array=w99, index=w98) -> (element=→"FilteredTrialData Display Channel":waveform(dbl))
          n246 = Index Array(array=w78, index (row)=w79) -> (element=→"NormalizedSignal1":dbl[])  [unwired: 1 in]
          n247 = Index Array(array=w78, index (row)=w80) -> (element=→"NormalizedSignal2":dbl[])  [unwired: 1 in]
          n248 = Index Array(array=w78, index (row)=w81) -> (element=→"NormalizedSignal3":dbl[])  [unwired: 1 in]
          n249 = Index Array(array=w78, index (row)=w82) -> (element=→"NormalizedSignal4":dbl[])  [unwired: 1 in]
          n250 = Index Array(array=w78, index (row)=w83) -> (element=→"NormalizedSignal5":dbl[])  [unwired: 1 in]
          n251 = Index Array(array=w78, index (row)=w84) -> (element=→"NormalizedSignal6":dbl[])  [unwired: 1 in]
          n252 = Index Array(array=w78, index (row)=w85) -> (element=→"NormalizedSignal7":dbl[])  [unwired: 1 in]
          n253 = Index Array(array=w78, index (row)=w86) -> (element=→"NormalizedSignal8":dbl[])  [unwired: 1 in]
          n254 = Index Array(array=w104, index=w101) -> (element=w76:dbl)
          "DisplayBarActivation" <- w76
          "DisplayActivation" <- w76
          n255 = call "FramesPerSecondTOMilliseconds.vi"("Thermometer\nFps"=w102) -> ("x*y"=w103:dbl)  [unwired: 10 in]
          n256 = Dequeue Element(queue=w75, error in (no error)=w74) -> (element=→"Raw Trial Data Wfm 2":waveform(dbl)[], error out=→"error out 3":errorcluster)  [unwired: 1 in, 2 out]
          n257 = Wait (ms)(milliseconds to wait=w103) -> ()  [unwired: 1 out]
          n258 = call "BarDisplay2Var.vi"("Activation Percentage"=w76, "Target Percentage"=w77) -> ()  [unwired: 10 in]
        }
        frame #2 {
          n259 = Tick Count (ms)() -> (millisecond timer value=w107:u32)
          n260 = Get Date/Time In Seconds() -> (seconds since 1Jan1904=→"End UI":timestamp)
          n261 = Subtract(x=w107, y=w106) -> (x-y=→"UI Elapsed Time":u32)
        }
      }
      n262 = local read "Reset"() -> (w64:bool)
    }
    n263 = disable-structure shown="Disabled" {
      frame Disabled {
        w48 = T4 4 items=["no dialog", "OK message", "continue or stop message", "OK message + warnings", "continue/stop + warnings"] ("type of dialog (OK msg:1)")
        w47 = 1 items=["no exception", "cancel error on match", "set error on match"] ("[exception action] (none:0)")
        w46 = 5 ("[exception code]")
        # "Save\nData\nFor\nVR"
        n264 = local read "UI Ampl Error Path"() -> (w49:path)
        n265 = local read "Amplitude Error"() -> (w50:dbl)
        n266 = local read "UI Percent Path"() -> (w55:path)
        n267 = local read "Target Percentage"() -> (w54:dbl)
        n268 = local read "UI Data Path"() -> (w61:path)
        n269 = local read "DisplayActivation"() -> (w59:dbl)
        n270 = Format Into String(w54) -> (resulting string=w56:string, error out=w57:errorcluster)  [unwired: 3 in]
        n271 = Format Into String(w50) -> (resulting string=w51:string, error out=w52:errorcluster)  [unwired: 3 in]
        n272 = Format Into String(w59) -> (resulting string=w60:string, error out=w62:errorcluster)  [unwired: 3 in]
        n273 = Write to Text File(file (use dialog)=w55, text=w56, error in=w57) -> (error out=w58:errorcluster)  [unwired: 1 in, 2 out]
        n274 = Write to Text File(file (use dialog)=w49, text=w51, error in=w52) -> (error out=w53:errorcluster)  [unwired: 1 in, 2 out]
        n275 = Write to Text File(file (use dialog)=w61, text=w60, error in=w62) -> (error out=w63:errorcluster)  [unwired: 1 in, 2 out]
        n276 = call <vilib>:"General Error Handler.vi"("type of dialog (OK msg:1)"=w48, "error in (no error)"=w63, "[exception action] (none:0)"=w47, "[exception code]"=w46) -> ()  [unwired: 7 in, 5 out]
        n277 = call <vilib>:"General Error Handler.vi"("type of dialog (OK msg:1)"=w48, "error in (no error)"=w58, "[exception action] (none:0)"=w47, "[exception code]"=w46) -> ()  [unwired: 7 in, 5 out]
        n278 = call <vilib>:"General Error Handler.vi"("type of dialog (OK msg:1)"=w48, "error in (no error)"=w53, "[exception action] (none:0)"=w47, "[exception code]"=w46) -> ()  [unwired: 7 in, 5 out]
      }
      frame Enabled {
      }
    }
  }
  n279 = Initialize Array(w12, 0 ("dimension size")) -> (→"Notes":cluster{timestamp, string}[])
  n280 = Bundle By Name("Y"=dbl[] []) -> (w35:waveform(dbl))  [unwired: 1 in]
  n281 = Initialize Array(0, 8 ("dimension size"), 0 ("dimension size")) -> (→"DisplayTrialData":i32[][])
  n282 = Initialize Array(w35, 8 ("dimension size")) -> (→"RawTrialData" →"FilteredDataArray":waveform(dbl)[])
  n283 = local read "MVC Window Size (s)"() -> (w5:dbl)
  n284 = local read "Display Window Size (s)"() -> (w3:dbl)
  n285 = local read "Sample rate (Hz)"() -> (w2:dbl)
  n286 = local read "Sample rate (Hz)"() -> (w6:dbl)
  n287 = Multiply(x=w6, y=w5) -> (x*y=w4:dbl)
  n288 = Multiply(x=w3, y=w2) -> (x*y=w1:dbl)
  n289 = Initialize Array(0.0 ("element"), 8 ("dimension size"), w4) -> (→"MVC Buffer":dbl[][])
  n290 = Initialize Array(0.0 ("element"), 8 ("dimension size"), w1) -> (→"Display Buffer":dbl[][])
  n291 = local write "MVCBufferSize"(w4) -> ()
  n292 = local write "DisplayBufferSize"(w1) -> ()
  n293 = Initialize Array(0.0 ("element"), 8 ("dimension size")) -> (→"MVCArray" →"DisplayValueByChannel":dbl[])
  n294 = local read "Sample rate (Hz)"() -> (w16:dbl)
  n295 = local read "Frames Per Second"() -> (w17:dbl)
  n296 = local read "Display Window Size (s)"() -> (w20:dbl)
  n297 = local read "Sample rate (Hz)"() -> (w19:dbl)
  n298 = local read "MVC Window Size (s)"() -> (w22:dbl)
  n299 = local read "Sample rate (Hz)"() -> (w24:dbl)
  n300 = Divide(x=w16, y=w17) -> (x/y=→"Samples per frame":dbl)
  n301 = Multiply(x=w22, y=w24) -> (x*y=→"MVCBufferSize":dbl)
  n302 = Multiply(x=w20, y=w19) -> (x*y=→"DisplayBufferSize":dbl)
  "Trial In Progress" <- FALSE ("Trial In Progress")
  "Get MVC" <- FALSE ("Acquiring Max")
  "Display Buffer Index" <- w13
  "Save MVC" <- FALSE ("Saving")
  "MVC Buffer Index" <- w13
  "Terminate" <- FALSE ("Terminate")
